vi "Configure Channel (Pulse Delta).vi"(0 "VISA resource name":refnum<visa-resource-name>, 1 "Enable Channel (True)":bool=TRUE, 2 "Range (0 : Level)":i32(ring) items=["Level", "Contact"], 3 "Chattering filter (On)":bool=TRUE, 4 "Span":T1={"Lower Span (-200000)"=-200000, "Upper Span (200000)"=200000} {"Upper Span (200000)" min=-200000 max=200000 step=1; "Lower Span (-200000)" min=-200000 max=200000 step=1}, 5 "error in (no error)":errorcluster, 6 "Channel (0001)":string="0001", 7 "Reference Channel (0001)":string="0001") -> (14 "VISA resource name out":refnum<visa-resource-name>, 15 "Channel":string, 19 "error out":errorcluster)   [LabVIEW 2020, in "Yokogawa GX Series.lvlib"]
doc: "Sets the input range of Pulse input channels.\n\nCommand: SRangePulse"
uses:
  <instrlib>/Yokogawa GX Series/Yokogawa GX Series.lvlib
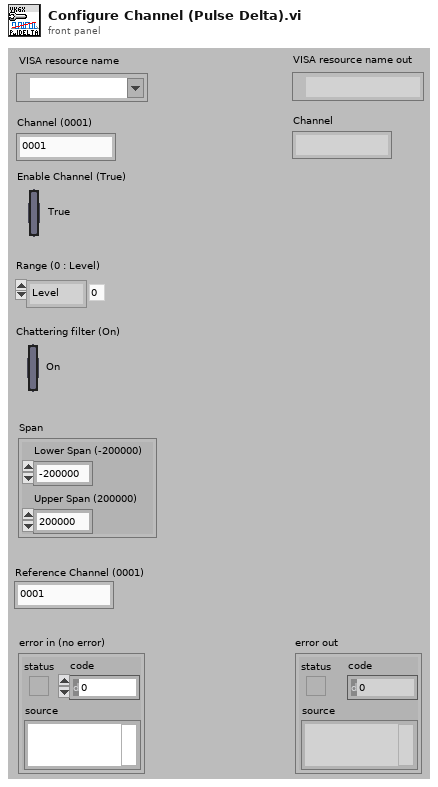
[diagram p1: front panel]
types:
  T1 = cluster{"Lower Span (-200000)":i32, "Upper Span (200000)":i32}
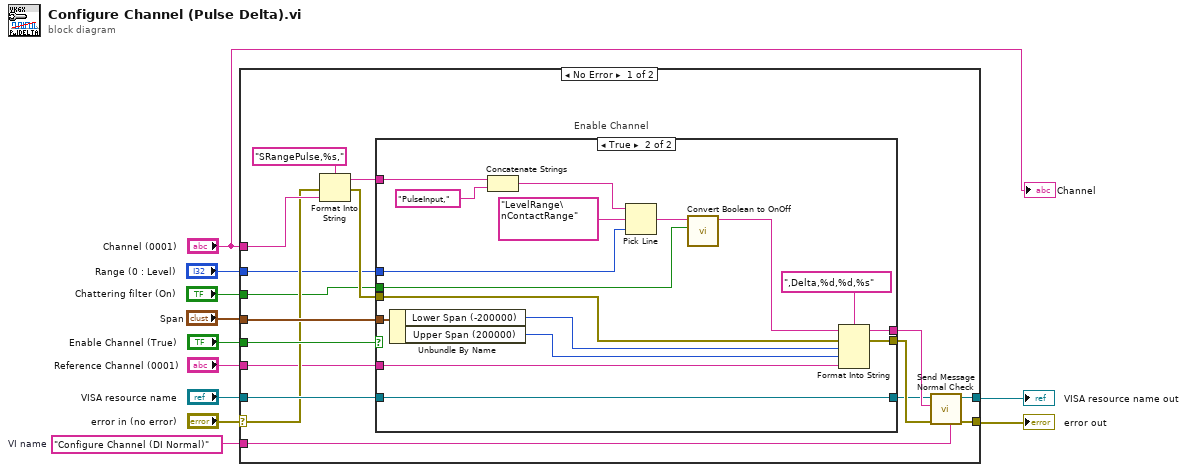
[diagram p0: block diagram]
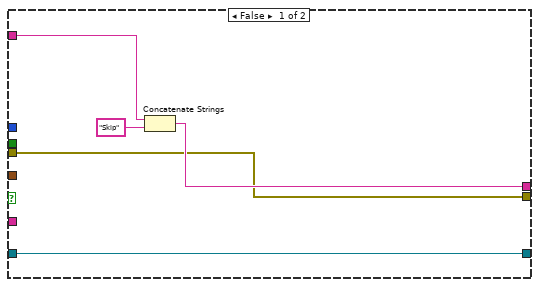
[diagram p2: hidden frame]
diagram:
  w8 = "Configure Channel (DI Normal)"  # VI name
  n1 = case shown="No Error" "error in (no error)" {
    selector: "error in (no error)" -> [w15 w51]
    tunnel: "Enable Channel (True)" -> [w25 _]
    tunnel: [w24 w52] -> w10
    tunnel: [w23 w51] -> w9
    tunnel: w8 -> [w20 _]
    tunnel: "Span" -> [w19 _]
    tunnel: "VISA resource name" -> [w18 w52]
    tunnel: "Channel (0001)" -> [w16 _]
    tunnel: "Range (0 : Level)" -> [w14 _]
    tunnel: "Chattering filter (On)" -> [w13 _]
    tunnel: "Reference Channel (0001)" -> [w12 _]
    frame No Error {
      # "Enable Channel"
      n2 = Format Into String(format string="SRangePulse,%s,", error in=w15, w16) -> (resulting string=w26:string, error out=w27:errorcluster)  [unwired: 1 in]
      n3 = case shown="True" w25 {
        tunnel: w27 -> [w30 w49]
        tunnel: [w30 w48] -> w22
        tunnel: w26 -> [w31 w42]
        tunnel: [w32 w47] -> w21
        tunnel: w19 -> [_ w46]
        tunnel: w18 -> [w29 w45]
        tunnel: [w29 w45] -> w17
        tunnel: w14 -> [_ w38]
        tunnel: w13 -> [_ w35]
        tunnel: w12 -> [_ w34]
        frame False {
          n4 = Concatenate Strings(w31, "Skip") -> (w32:string)
        }
        frame True {
          n5 = Unbundle By Name(w46) -> ("Lower Span (-200000)"=w44:i32, "Upper Span (200000)"=w43:i32)
          n6 = Concatenate Strings(w42, "PulseInput,") -> (w40:string)
          n7 = Pick Line(string ("")=w40, multi-line string="LevelRange\nContactRange", line index=w38) -> (output string=w37:string)
          n8 = call <instrlib>:"Convert Boolean to OnOff.vi"("On/Off"=w35, "Initial String (\"\")"=w37) -> ("Resulting String"=w36:string)  [unwired: 9 in]
          n9 = Format Into String(format string=",Delta,%d,%d,%s", initial string=w36, error in=w49, w44, w43, w34) -> (resulting string=w47:string, error out=w48:errorcluster)
        }
      }
      n10 = call <instrlib>:"Send Message Normal Check.vi"("Source (\"\")"=w20, "error in (no error)"=w22, "Send Message (\"\")"=w21, "VISA resource name"=w17) -> ("error out"=w23:errorcluster, "VISA resource name out"=w24:refnum<visa-resource-name>)  [unwired: 2 in, 4 out]
    }
    frame Error {
    }
  }
  "error out" <- w9
  "VISA resource name out" <- w10
  "Channel" <- "Channel (0001)"
